vi "CSVlog - Kapcsolásra CSV-be mentés.vi"() -> ()   [LabVIEW 2020]
uses:
  <vilib>/Utility/file.llb/Write Delimited Spreadsheet (string).vi
panel:
  in  "stop":bool
  in  "Boolean":bool
  in  "file path (dialog if empty)":path
  in  "Cluster":cluster{"Numeric":dbl, "String":string}
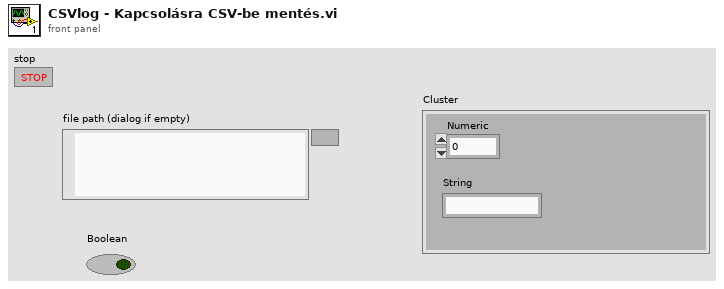
[diagram p1: front panel]
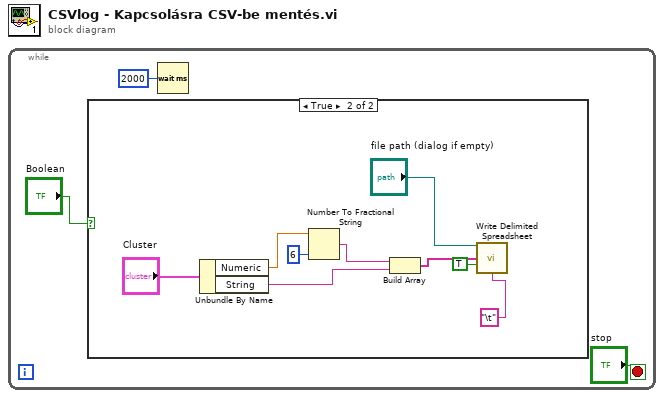
[diagram p0: block diagram]
diagram:
  n1 = while {
    stop <- "stop" stop-if-true
    n2 = case shown="True" "Boolean" {
      frame False {
      }
      frame True {
        n3 = Unbundle By Name("Cluster") -> ("Numeric"=w8:dbl, "String"=w10:string)
        n4 = Number To Fractional String(number=w8, precision (6)=i16 6) -> (F-format string=w9:string)  [unwired: 2 in]
        n5 = Build Array(w9, w10) -> (w11:string[])
        n6 = call-poly <vilib>:"Write Delimited Spreadsheet.vi"("file path (dialog if empty)"="file path (dialog if empty)", "1D data"=w11, "append to file? (new file:F)"=TRUE, "delimiter (\\t)"="\t" ("delimiter (\\t)")) -> ()  [unwired: 10 in, 2 out]
      }
    }
    n7 = Wait (ms)(milliseconds to wait=u32 2000) -> ()  [unwired: 1 out]
  }
